vi "goStraighbool.vi"(8 "error in (no error)":errorcluster, 9 "Robot - Ball":dbl[](array[numeric]) format="%0.2f", 10 "Ball - Target":dbl[](array[numeric]) format="%0.2f", 11 "KickToSkill in":refnum<class "KickToSkill.lvclass">) -> (0 "error out":errorcluster, 2 "go straight?":bool, 3 "KickToSkill out":refnum<class "KickToSkill.lvclass">)   [LabVIEW 2021, in "KickToSkill.lvclass"]
uses:
  KickToSkill.lvclass
  Game_class/Game.lvclass
  <vilib>/Analysis/coordinate.llb/2D Cartesian Coordinate Rotation (Scalar).vi
  <vilib>/Analysis/NI_AALPro.lvlib
panel:
  in  "Game":refnum<class "Game.lvclass">
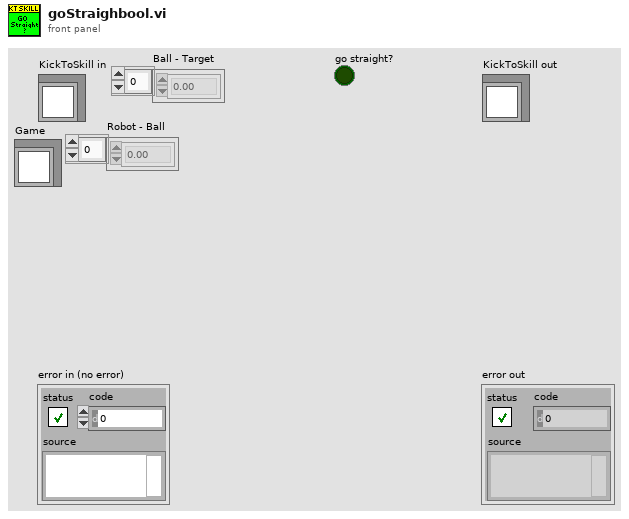
[diagram p1: front panel]
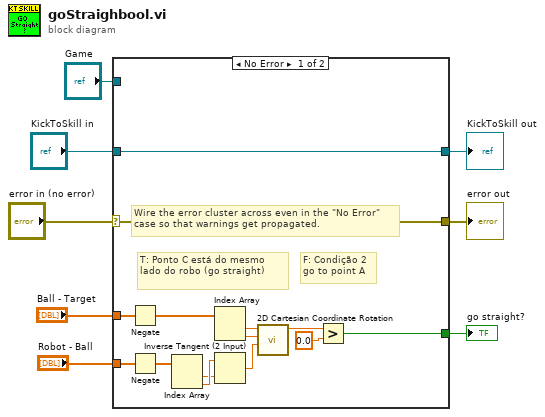
[diagram p0: block diagram]
diagram:
  n1 = case shown="No Error" "error in (no error)" {
    selector: "error in (no error)" -> [w22 w24]
    tunnel: [w22 w24] -> w7
    tunnel: [w21 w23] -> w5
    tunnel: "KickToSkill in" -> [w21 w23]
    tunnel: "Game" -> [_ _]
    tunnel: [w11 _] -> w3
    tunnel: "Ball - Target" -> [w10 _]
    tunnel: "Robot - Ball" -> [w9 _]
    frame No Error {
      # "F: Condição 2\ngo to point A"
      # "T: Ponto C está do mesmo lado do robo (go straight)"
      # "Wire the error cluster across even in the \"No Error\"\ncase so that warnings get propagated."
      n2 = Negate(x=w10) -> (-x=w13:dbl[])
      n3 = Negate(x=w9) -> (-x=w12:dbl[])
      n4 = Index Array(array=w12) -> (element #1=w15:dbl, element #2=w16:dbl)  [unwired: 2 in]
      n5 = Index Array(array=w13) -> (element #1=w17:dbl, element #2=w18:dbl)  [unwired: 2 in]
      n6 = Inverse Tangent (2 Input)(1:w15, 2:w16) -> (0:w14:dbl)
      n7 = call-poly <vilib>:"2D Cartesian Coordinate Rotation.vi"("theta"=w14, "y"=w18, "x"=w17) -> ("x out"=w19:dbl)  [unwired: 6 in, 2 out]
      n8 = Greater?(x=w19, y=0.0) -> (0:w11:bool)
    }
    frame Error {
    }
  }
  "error out" <- w7
  "KickToSkill out" <- w5
  "go straight?" <- w3
